vi "Check existence.vi"(6 "Type":enum16{"Column & Table", "Table", "Column"}(ring), 8 "error in (no error)":errorcluster, 9 "Column Name":string, 10 "Table Name":string, 11 "Data.PG":refnum<class "LV-Data.PGSQL.lvclass">) -> (0 "error out":errorcluster, 2 "Exists?":bool, 3 "Data.PG out":refnum<class "LV-Data.PGSQL.lvclass">)   [LabVIEW 2019, in "LV-Data.PGSQL.lvclass"]
uses:
  LV-Data.PGSQL.lvclass
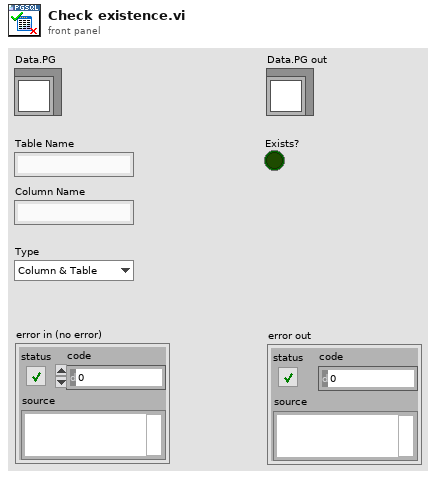
[diagram p1: front panel]
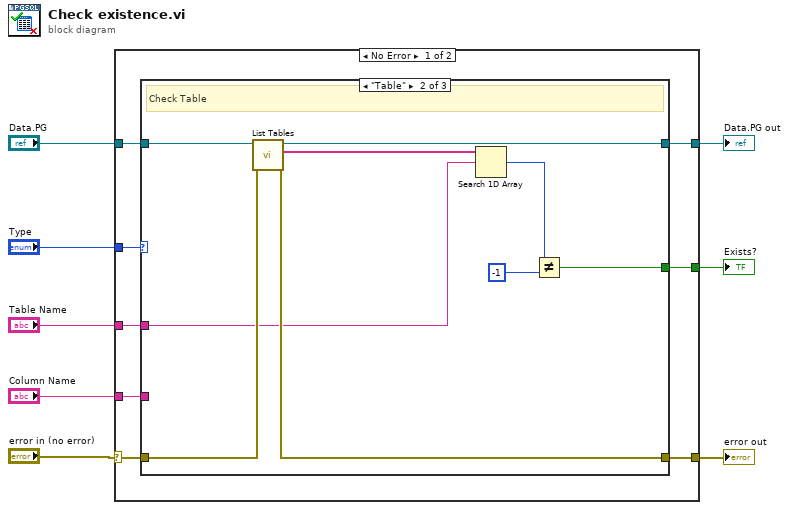
[diagram p0: block diagram]
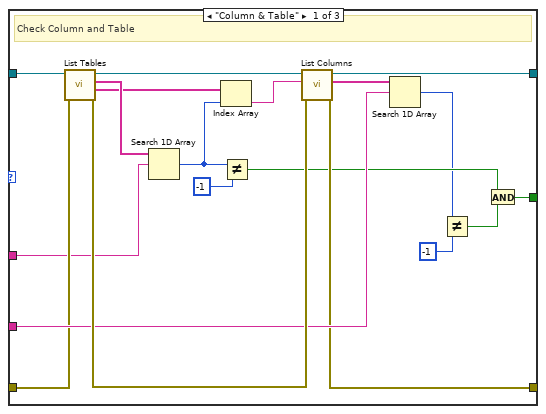
[diagram p2: hidden frame]
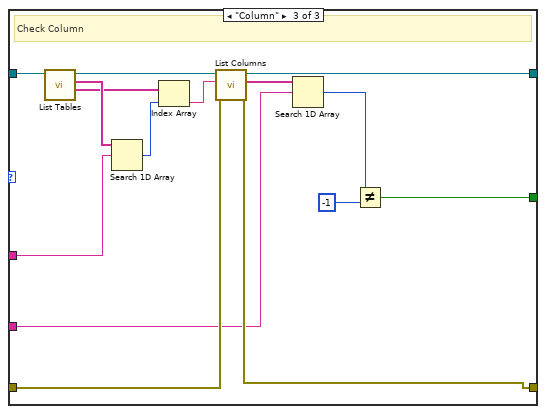
[diagram p3: hidden frame]
diagram:
  n1 = case shown="No Error" "error in (no error)" {
    selector: "error in (no error)" -> [w9 w61]
    tunnel: "Type" -> [w16 _]
    tunnel: "Data.PG" -> [w15 w60]
    tunnel: "Table Name" -> [w14 _]
    tunnel: [w13 _] -> w5
    tunnel: [w12 w60] -> w4
    tunnel: [w11 w61] -> w3
    tunnel: "Column Name" -> [w10 _]
    frame No Error {
      n2 = case shown="\"Table\"" w16 {
        tunnel: w15 -> [w35 w44 w51]
        tunnel: w9 -> [w28 w42 w58]
        tunnel: w14 -> [w26 w39 w49]
        tunnel: [w31 w38 w55] -> w13
        tunnel: [w29 w43 w59] -> w12
        tunnel: [w30 w41 w57] -> w11
        tunnel: w10 -> [w32 _ w54]
        frame "Column & Table" {
          # "Check Column and Table"
          n3 = call "List Tables.vi"("error in (no error)"=w28, "Data.PG"=w35) -> ("error out"=w33:errorcluster, "Table Paths"=w20:string[], "Table Names"=w21:string[], "Data.PG"=w34:refnum<class "LV-Data.PGSQL.lvclass">)  [unwired: 6 in]
          n4 = Search 1D Array(1D array=w21, element=w26) -> (index of element=w19:i32)  [unwired: 1 in]
          n5 = Index Array(array=w20, index=w19) -> (element=w18:string)
          n6 = Not Equal?(x=w19, y=-1) -> (x != y?=w25:bool)
          n7 = call "List Columns.vi"("error in (no error)"=w33, "Table Path"=w18, "Data.PG"=w34) -> ("error out"=w30:errorcluster, "Column Names"=w27:string[], "Data.PG out"=w29:refnum<class "LV-Data.PGSQL.lvclass">)  [unwired: 4 in, 2 out]
          n8 = Search 1D Array(1D array=w27, element=w32) -> (index of element=w17:i32)  [unwired: 1 in]
          n9 = Not Equal?(x=w17, y=-1) -> (x != y?=w24:bool)
          n10 = And(x=w25, y=w24) -> (x .and. y?=w31:bool)
        }
        frame "Table" {
          # "Check Table"
          n11 = call "List Tables.vi"("error in (no error)"=w42, "Data.PG"=w44) -> ("error out"=w41:errorcluster, "Table Names"=w36:string[], "Data.PG"=w43:refnum<class "LV-Data.PGSQL.lvclass">)  [unwired: 6 in, 1 out]
          n12 = Search 1D Array(1D array=w36, element=w39) -> (index of element=w37:i32)  [unwired: 1 in]
          n13 = Not Equal?(x=w37, y=-1) -> (x != y?=w38:bool)
        }
        frame "Column" {
          # "Check Column"
          n14 = call "List Tables.vi"("Data.PG"=w51) -> ("Table Paths"=w47:string[], "Table Names"=w48:string[], "Data.PG"=w50:refnum<class "LV-Data.PGSQL.lvclass">)  [unwired: 7 in, 1 out]
          n15 = Search 1D Array(1D array=w48, element=w49) -> (index of element=w46:i32)  [unwired: 1 in]
          n16 = Index Array(array=w47, index=w46) -> (element=w45:string)
          n17 = call "List Columns.vi"("error in (no error)"=w58, "Table Path"=w45, "Data.PG"=w50) -> ("error out"=w57:errorcluster, "Column Names"=w53:string[], "Data.PG out"=w59:refnum<class "LV-Data.PGSQL.lvclass">)  [unwired: 4 in, 2 out]
          n18 = Search 1D Array(1D array=w53, element=w54) -> (index of element=w52:i32)  [unwired: 1 in]
          n19 = Not Equal?(x=w52, y=-1) -> (x != y?=w55:bool)
        }
      }
    }
    frame Error {
    }
  }
  "Exists?" <- w5
  "Data.PG out" <- w4
  "error out" <- w3
